vi "Create.vi"(8 "error in (no error)":errorcluster, 10 "size":i32, 11 "name":string) -> (0 "error out":errorcluster, 3 "reference":T1)   [LabVIEW 2017, in "DVRBuffer.lvlib"]
uses:
  <vilib>/addons/InsightCM/Devices/Shared/Common/DVRBuffer/DVRBuffer.lvlib
  <vilib>/addons/PointValueMap/controls/PointMap.ctl
  <vilib>/addons/InsightCM/Devices/Shared/Common/DVRBuffer/controls/DVRElement.ctl
  <vilib>/addons/InsightCM/Devices/Shared/Common/DVRBuffer/controls/DVRBuffer.ctl
  <vilib>/addons/PointValueMap/subVIs/Point_Write_variant.vi
  <vilib>/addons/PointValueMap/PointValueMap.lvlib
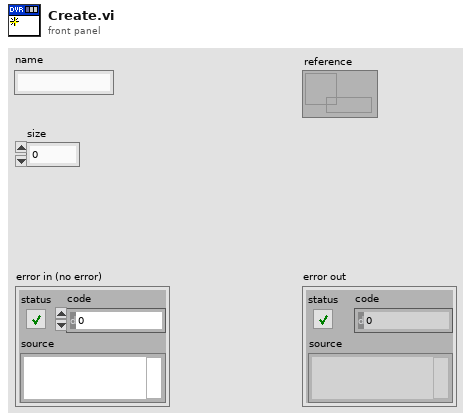
[diagram p1: front panel]
types:
  T1 = typedef "PointValueMap.lvlib/PointMap.ctl" = refnum<data-value>
  T2 = typedef "DVRBuffer.lvlib/DVRBuffer.ctl" = cluster{"buffer":T3[], "write ptr index":i32, "last block":u32, "buffer size":u32}
  T3 = typedef "DVRBuffer.lvlib/DVRElement.ctl" = cluster{"location":u32, "DVR":u32, "points":i32, "dt":dbl, "PulsePositions":dbl[], "Pulses Per Rev":dbl}
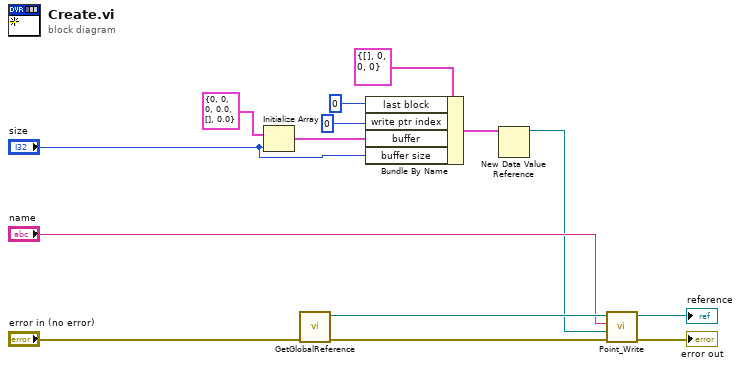
[diagram p0: block diagram]
diagram:
  n1 = Initialize Array(T3 {"location"=0, "DVR"=0, "points"=0, "dt"=0.0, "PulsePositions"=[], "Pulses Per Rev"=0.0}, "size") -> (w8:T3[])
  n2 = call <vilib>:"GetGlobalReference.vi"("error in (no error)"="error in (no error)") -> ("error out"=w13:errorcluster, "reference"=w12:T1)  [unwired: 9 in]
  n3 = Bundle By Name(cluster=T2 {"buffer"=[], "write ptr index"=0, "last block"=0, "buffer size"=0} ("DVRBuffer"), "last block"=u32 0 ("write ptr monotonic"), "write ptr index"=0, "buffer"=w8, "buffer size"="size") -> (w5:T2)
  n4 = New Data Value Reference(data value=w5) -> (data value reference=w4:refnum<data-value>)  [unwired: 1 in, 1 out]
  n5 = call-poly <vilib>:"Point_Write.vi"("Error In"=w13, "Value"=w4, "Tag"="name", "Map"=w12) -> ("Error Out"=→"error out":errorcluster, "Map Out"=→"reference":T1)  [unwired: 6 in]
